vi "1.Basic demo.vi"() -> ()   [LabVIEW 2023]
uses:
  C:/Users/fg/Documents/UniversalRobots.vi/UnderAutomation.UniversalRobots/lib/UnderAutomation.UniversalRobots.dll
  UnderAutomation.UniversalRobots/lib/UnderAutomation.UniversalRobots.dll
  UnderAutomation.UniversalRobots/UnderAutomation.UniversalRobots.lvlib
panel:
  out "Configurable0":bool
  out "error out":errorcluster
  out "Waveform 1":dbl(graph)
  out "Connected":bool
  in  "stop":bool
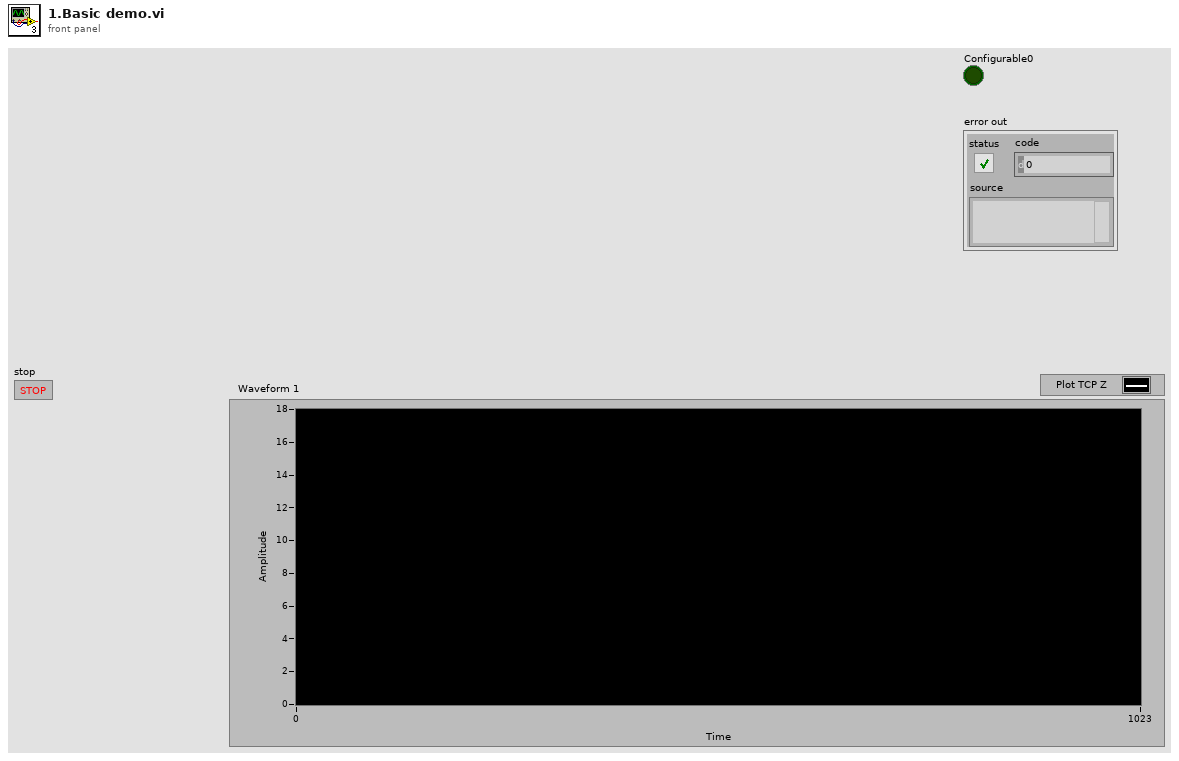
[diagram p1: front panel]
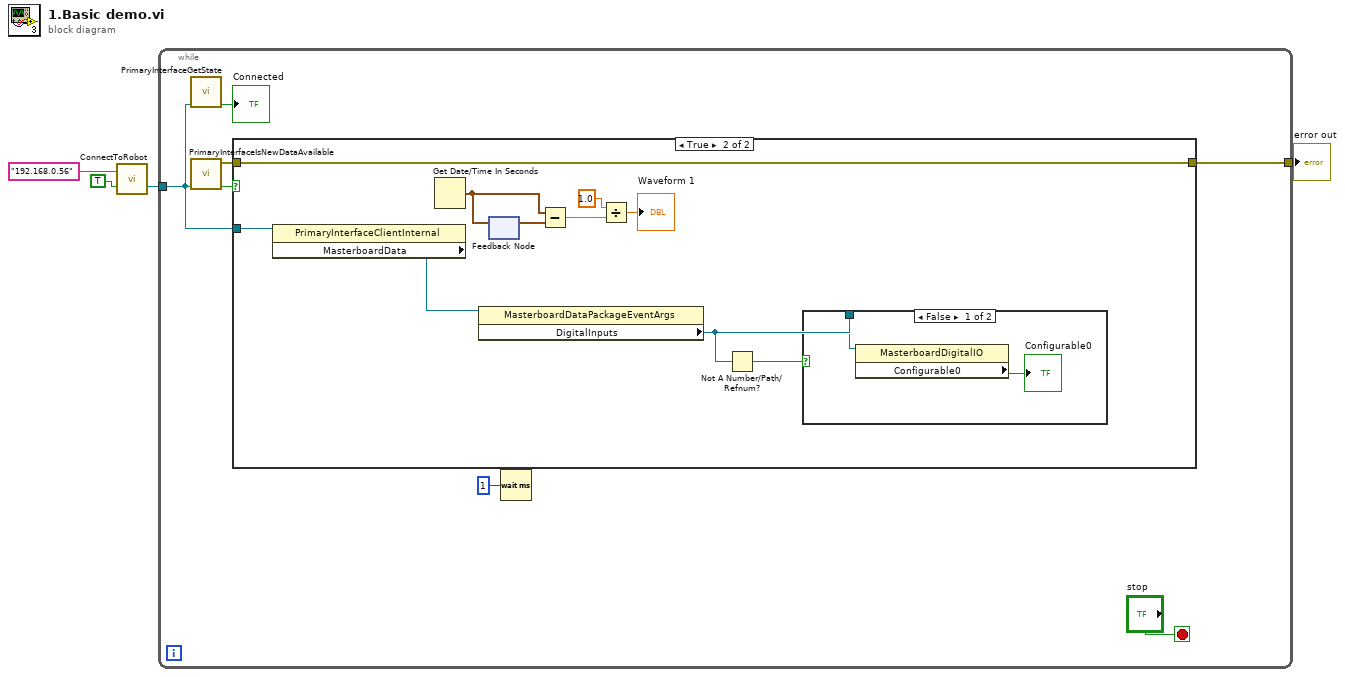
[diagram p0: block diagram]
diagram:
  n1 = call "ConnectToRobot.vi"("ip"="192.168.0.56", "Enable Primary Interface"=TRUE) -> ("PrimaryInterface"=w1:refnum<k24>)  [unwired: 13 in, 4 out]
  n2 = while {
    tunnel: w1 -> [w7]
    tunnel: [w5] -> w2
    stop <- "stop" stop-if-true
    n3 = call "PrimaryInterfaceGetState.vi"("PrimaryInterface"=w7) -> ("Connected"=→"Connected":bool)  [unwired: 9 in, 1 out]
    n4 = call "PrimaryInterfaceIsNewDataAvailable.vi"("PrimaryInterface"=w7) -> ("Data available"=w8:bool, "error out"=w6:errorcluster)  [unwired: 9 in]
    n5 = case shown="True" w8 {
      tunnel: w7 -> [_ w17]
      tunnel: w6 -> [w12 w15]
      tunnel: [w12 w15] -> w5
      frame False {
      }
      frame True {
        n6 = property class="PrimaryInterfaceClientInternal"(reference=w17) -> ("MasterboardData"=w16:refnum<k24>)  [unwired: 1 in, 2 out]
        n7 = Get Date/Time In Seconds() -> (seconds since 1Jan1904=w22:timestamp)
        n8 = property class="MasterboardDataPackageEventArgs"(reference=w16) -> ("DigitalInputs"=w13:refnum<k24>)  [unwired: 1 in, 2 out]
        n9 = feedback #1() -> (w21:timestamp)  [unwired: 1 in]
        n10 = feedback-in #1(w22) -> ()
        n11 = Subtract(x=w22, y=w21) -> (x-y=w20:dbl)
        n12 = Divide(x=1.0, y=w20) -> (x/y=→"Waveform 1":dbl)
        n13 = Not A Number/Path/Refnum?(number/path/refnum=w13) -> (NaN/Path/Refnum?=w14:bool)
        n14 = case shown="False" w14 {
          tunnel: w13 -> [w24 _]
          frame False {
            n15 = property class="MasterboardDigitalIO"(reference=w24) -> ("Configurable0"=→"Configurable0":bool)  [unwired: 1 in, 2 out]
          }
          frame True {
          }
        }
      }
    }
    n16 = Wait (ms)(milliseconds to wait=u32 1) -> ()  [unwired: 1 out]
  }
  "error out" <- w2
